vi "Process Measurement.vi"(0 "Waveform":waveform(dbl), 5 "NoEdges":i32, 11 "error in":errorcluster) -> (4 "Test Values":T1, 15 "error out":errorcluster)   [LabVIEW 2023, in "AI.lvlib"]
uses:
  AI.lvlib
  Test Values.ctl
  <vilib>/measure/mascope.llb/Amplitude and Levels 1 chan.vi
  <vilib>/measure/mascope.llb/Transition Measurements 1 chan.vi
  <vilib>/measure/NI_MAPro.lvlib
panel:
  out "Rise values":dbl[](array[numeric])
  out "Fall values":dbl[](array[numeric])
  out "low state level":dbl format="%.2g"
  out "high state level":dbl format="%.2g"
  out "Rise time":dbl
  out "Fall time":dbl
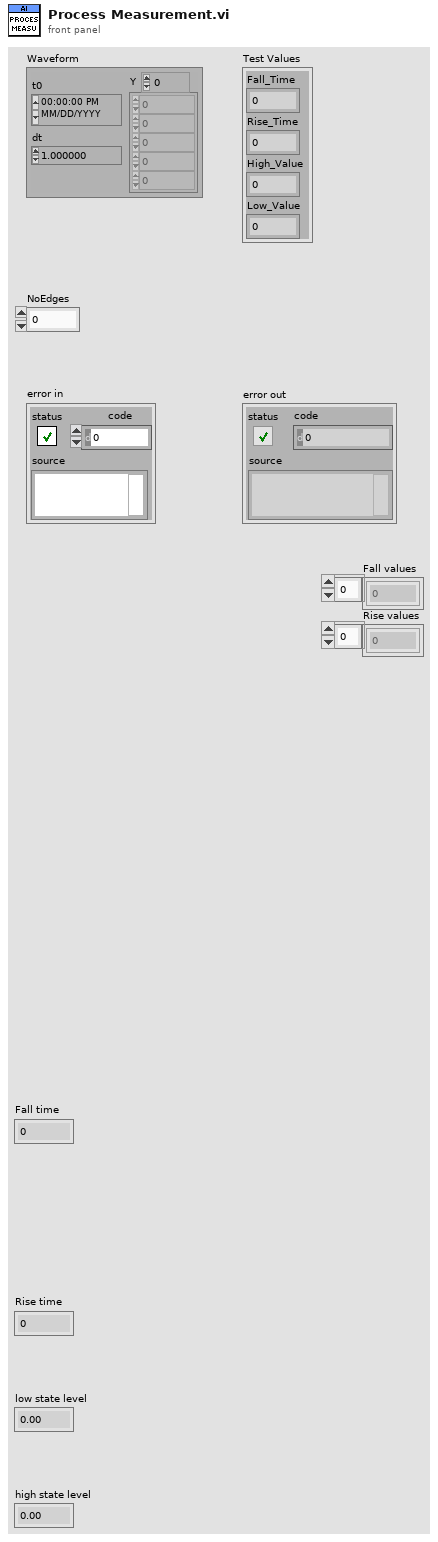
[diagram p1: front panel]
types:
  T1 = typedef "AI.lvlib/Test Values.ctl" = cluster{"Fall_Time":dbl, "Rise_Time":dbl, "High_Value":dbl, "Low_Value":dbl}
  T2 = cluster{"high ref level":dbl, "mid ref level":dbl, "low ref level":dbl, "ref units":u16}
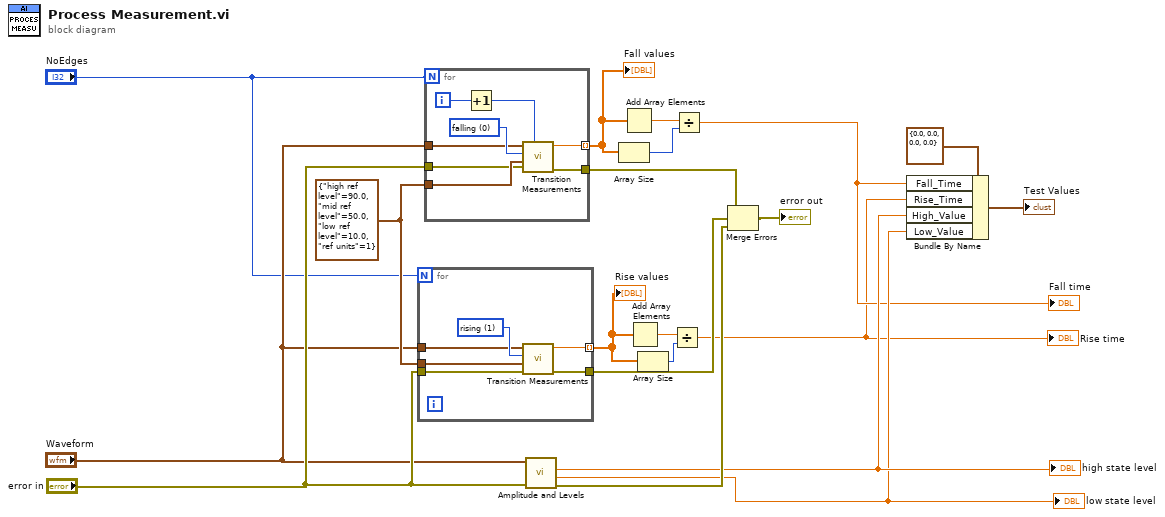
[diagram p0: block diagram]
diagram:
  w20 = T2 {"high ref level"=90.0, "mid ref level"=50.0, "low ref level"=10.0, "ref units"=1} ("reference levels")
  n1 = for {
    N: "NoEdges" -> [_]
    tunnel: w20 -> [w25]
    tunnel: [w22] -> w4 mode=indexing
    tunnel: "Waveform" -> [w21]
    tunnel: "error in" -> [w24]
    tunnel: [w23] -> w17
    w26 = u16 1 items=["falling", "rising"] ("polarity (rising)")
    n2 = call-poly <vilib>:"Transition Measurements.vi"("error in (no error)"=w24, "reference levels"=w25, "polarity (rising)"=w26, "signal in"=w21) -> ("error out"=w23:errorcluster, "transition duration"=w22:dbl)  [unwired: 2 in, 4 out]
  }
  "Rise values" <- w4
  n3 = for {
    N: "NoEdges" -> [_]
    tunnel: w20 -> [w33]
    tunnel: [w30] -> w6 mode=indexing
    tunnel: "Waveform" -> [w29]
    tunnel: "error in" -> [w32]
    tunnel: [w31] -> w18
    i -> [w28]
    w34 = u16 0 items=["falling", "rising"] ("polarity (rising)")
    n4 = Increment(x=w28) -> (x+1=w27:i32)
    n5 = call-poly <vilib>:"Transition Measurements.vi"("edge number (1)"=w27, "error in (no error)"=w32, "reference levels"=w33, "polarity (rising)"=w34, "signal in"=w29) -> ("error out"=w31:errorcluster, "transition duration"=w30:dbl)  [unwired: 1 in, 4 out]
  }
  "Fall values" <- w6
  n6 = call-poly <vilib>:"Amplitude and Levels.vi"("error in (no error)"="error in", "signal in"="Waveform") -> ("error out"=w16:errorcluster, "low state level"=w12:dbl, "high state level"=w13:dbl)  [unwired: 6 in, 1 out]
  "high state level" <- w13
  "low state level" <- w12
  n7 = Array Size(array=w6) -> (size(s)=w5:i32)
  n8 = Add Array Elements(numeric array=w6) -> (sum=w8:dbl)
  n9 = Add Array Elements(numeric array=w4) -> (sum=w3:dbl)
  n10 = Array Size(array=w4) -> (size(s)=w2:i32)
  n11 = Divide(x=w3, y=w2) -> (x/y=w1:dbl)
  "Rise time" <- w1
  n12 = Divide(x=w8, y=w5) -> (x/y=w7:dbl)
  "Fall time" <- w7
  n13 = Merge Errors(w18, w17, w16) -> (→"error out":errorcluster)
  n14 = Bundle By Name(cluster=T1 {"Fall_Time"=0.0, "Rise_Time"=0.0, "High_Value"=0.0, "Low_Value"=0.0}, "Fall_Time"=w7, "Rise_Time"=w1, "High_Value"=w13, "Low_Value"=w12) -> (→"Test Values":T1)
